vi "Safety Trigger.vi"(8 "error in (no error)":errorcluster) -> (0 "error out":errorcluster)   [LabVIEW 2019, in "Haptic Prog Interface.lvlib"]
doc: "Returns the forces of the haptic pen in N.\n\n<b>Position:</b> Returns a cluster of the x, y, and z forces on the pen (in units of N)."
uses:
  Haptic Prog Interface.lvlib
  dll_path.vi
panel:
  out "Trigger State":bool
  in  "Safety Trigger":bool
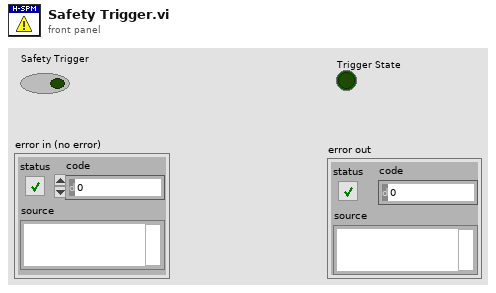
[diagram p1: front panel]
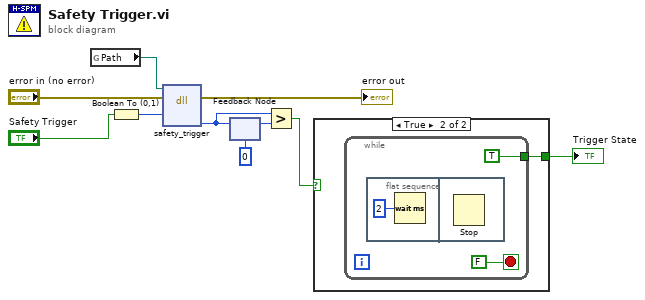
[diagram p0: block diagram]
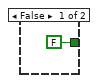
[diagram p2: hidden frame]
diagram:
  n1 = global read "dll_path.vi" "Path"() -> (w10:path)
  n2 = Boolean To (0,1)(Boolean="Safety Trigger") -> (0, 1=w7:i16)
  n3 = dll-call lib="C:/Users/freem/Documents/GitHub/HapticSPM/Haptic-Programming-Interface/x64/Debug/Haptic Programming Interface.dll" fn="safety_trigger"(path in=w10, error in="error in (no error)", "input"=w7) -> (error out=→"error out":errorcluster, "output"=w1:i32)  [unwired: 4 in, 1 out]
  n4 = feedback-in #1(w1) -> ()
  n5 = feedback #1(0) -> (w4:i32)
  n6 = Greater?(x=w1, y=w4) -> (0:w3:bool)
  n7 = case shown="True" w3 {
    tunnel: [FALSE w12] -> w2
    frame False {
    }
    frame True {
      n8 = while {
        tunnel: [TRUE] -> w12
        stop <- FALSE stop-if-true
        n9 = flat-sequence {
          frame #0 {
            n10 = Wait (ms)(milliseconds to wait=u32 2) -> ()  [unwired: 1 out]
          }
          frame #1 {
            n11 = Stop() -> ()  [unwired: 1 in]
          }
        }
      }
    }
  }
  "Trigger State" <- w2
